vi ".out Path.vi"(0 "Enable":bool=TRUE, 5 "error in (no error)":errorcluster) -> (17 "Path":string, 18 "OK":bool, 19 "error out":errorcluster)   [LabVIEW 2017]
doc: "Displays a standard dialog box that prompts users to enter information, such as a user name and password.\n--------------------\n\nThis Express VI is configured as follows:\n\nMessage to Display to the User:Please select the path\nThe inputs are: \nText Entry Box: Path"
panel:
  in  "Path":path
  out "String":string="Please select the path"
  in  "Cancel":bool
  in  "OK2":bool
  in  "OK1":bool
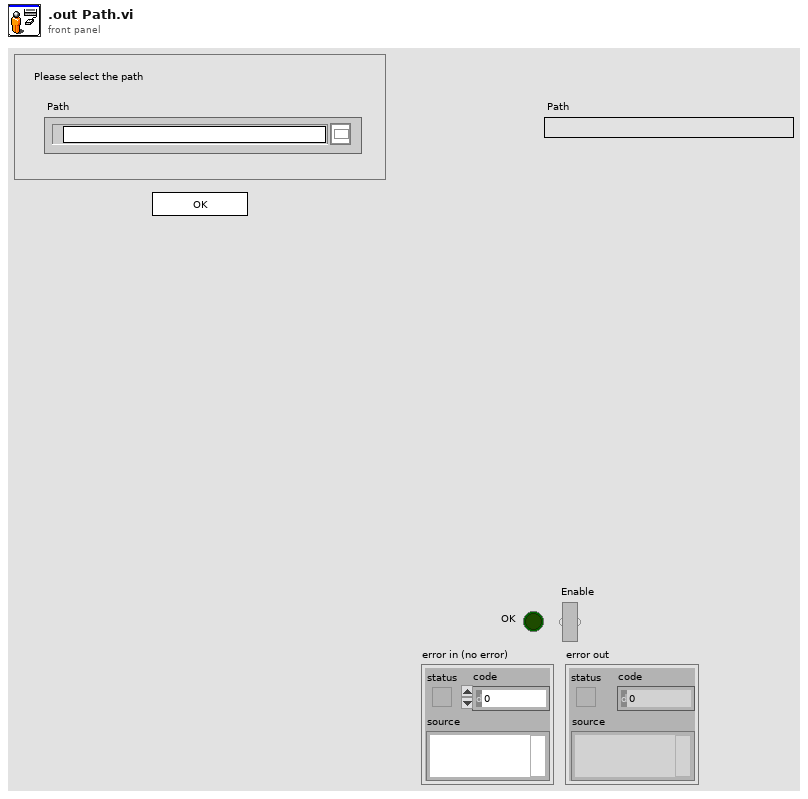
[diagram p1: front panel]
types:
  T1 = cluster{"Input Name":string, "Input Data Type":i32}[]
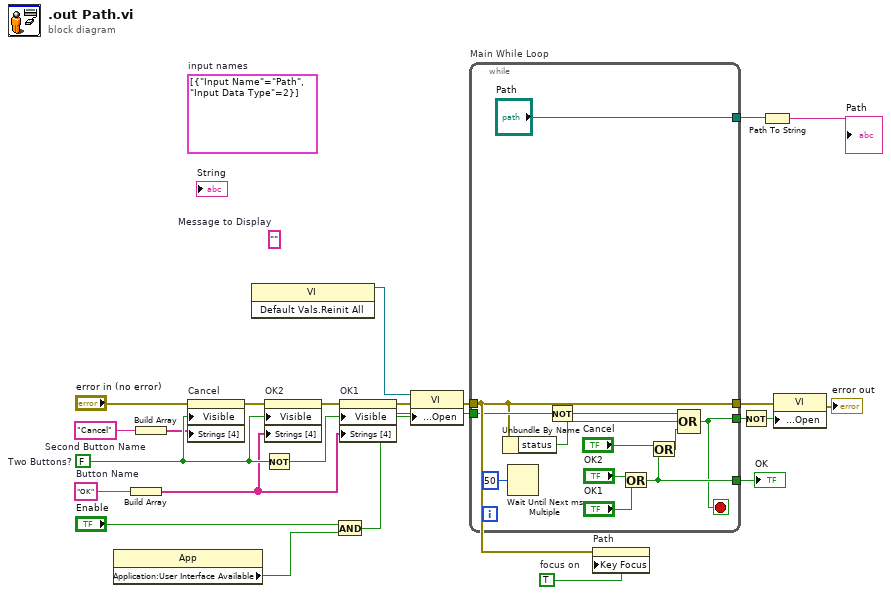
[diagram p0: block diagram]
diagram:
  w3 = TRUE  # focus on
  (unwired) T1 [{"Input Name"="Path", "Input Data Type"=2}]  # input names
  w15 = "Cancel"  # Second Button Name
  w13 = "OK"  # Button Name
  (unwired) ""  # Message to Display
  w23 = FALSE  # Two Buttons?
  n1 = property class="App"() -> ("Application:User Interface Available"=w5:bool)  [unwired: 2 in, 2 out]
  n2 = Build Array(w13) -> (w14:string[])
  n3 = Build Array(w15) -> (w16:string[])
  n4 = property on="Cancel" class="Bool"(error in="error in (no error)", "Visible"=w23, "Strings [4]"=w16) -> (error out=w20:errorcluster)  [unwired: 1 in, 1 out]
  n5 = invoke class="VI" method="Default Vals.Reinit All"() -> (reference out=w4:refnum<vi>)  [unwired: 3 in, 2 out]
  n6 = Not(x=w23) -> (.not. x?=w21:bool)
  n7 = property on="OK2" class="Bool"(error in=w20, "Visible"=w23, "Strings [4]"=w14) -> (error out=w19:errorcluster)  [unwired: 1 in, 1 out]
  n8 = And(x="Enable", y=w5) -> (x .and. y?=w6:bool)
  n9 = property on="OK1" class="Bool"(error in=w19, "Visible"=w21, "Strings [4]"=w14) -> (error out=w12:errorcluster)  [unwired: 1 in, 1 out]
  n10 = property class="VI"(reference=w4, error in=w12, "Front Panel Window:Open"=w6) -> (error out=w11:errorcluster)  [unwired: 1 out]
  n11 = while "Main While Loop" {
    tunnel: [w32] -> w22
    tunnel: w6 -> [w30]
    tunnel: [w28] -> w17
    tunnel: w11 -> [w27]
    tunnel: [w27] -> w9
    tunnel: ["Path"] -> w2
    stop <- w28 stop-if-true
    n12 = Unbundle By Name(w27) -> ("status"=w25:bool)
    n13 = Wait Until Next ms Multiple(millisecond multiple=u32 50) -> ()  [unwired: 1 out]
    n14 = Not(x=w30) -> (.not. x?=w29:bool)
    n15 = Or(x="OK2", y="OK1") -> (x .or. y?=w32:bool)
    n16 = Or(x="Cancel", y=w32) -> (x .or. y?=w26:bool)
    n17 = Compound Arithmetic op=OR(w29, w25, w26) -> (w28:bool)
  }
  "OK" <- w22
  n18 = property on="Path" class="Path"(error in=w11, "Key Focus"=w3) -> ()  [unwired: 1 in, 2 out]
  n19 = Not(x=w17) -> (.not. x?=w18:bool)
  n20 = Path To String(path=w2) -> (string=→"Path":string)
  n21 = property class="VI"(error in=w9, "Front Panel Window:Open"=w18) -> (error out=→"error out":errorcluster)  [unwired: 1 in, 1 out]
